vi "GV TriggerAODOexternal.vi"() -> ()   [LabVIEW 2017]
panel:
  out "TriggerAODOexternal":bool
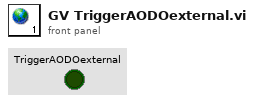
[diagram p1: front panel]
diagram:
